vi "SelfParking.vi"() -> ()   [LabVIEW 2020]
uses:
  <vilib>/Instr/_visa.llb/VISA Flush IO Buffer Mask.ctl
  <vilib>/Instr/_visa.llb/VISA Configure Serial Port (Instr).vi
panel:
  out "Ask user":bool
  out "Perpendicular":bool
  out "Parallel":bool
  out "Execute":bool
  out "Move to stop line":bool
  out "Wait for start":bool
  out "Ask user":bool
  out "Scanning":bool
  out "String":string
  in  "module path":path
  in  "stop 2":bool
  in  "stop":bool
  out "Centimeters":i32
  in  "VISA resource name":refnum<visa-resource-name>
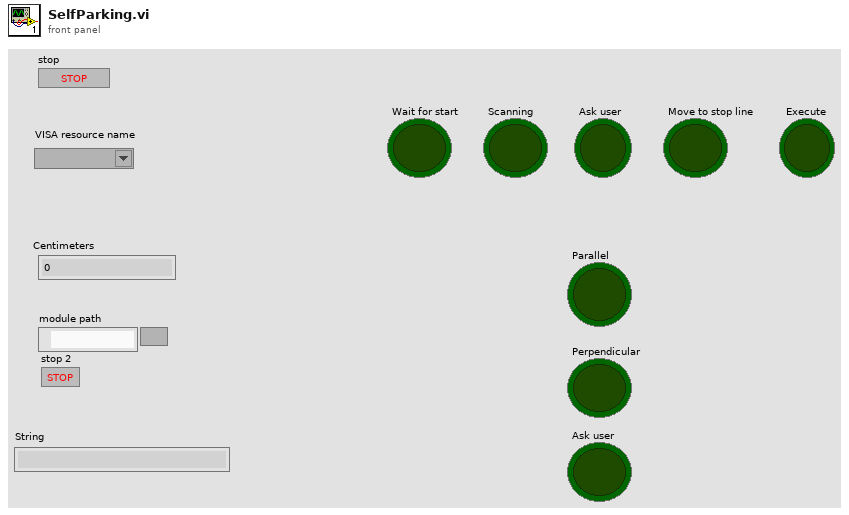
[diagram p1: front panel]
types:
  T1 = enum16{"wait for start", "move to stop line", "scanning", "ask user", "execute park"}
  T2 = typedef "VISA Flush IO Buffer Mask.ctl" = u16
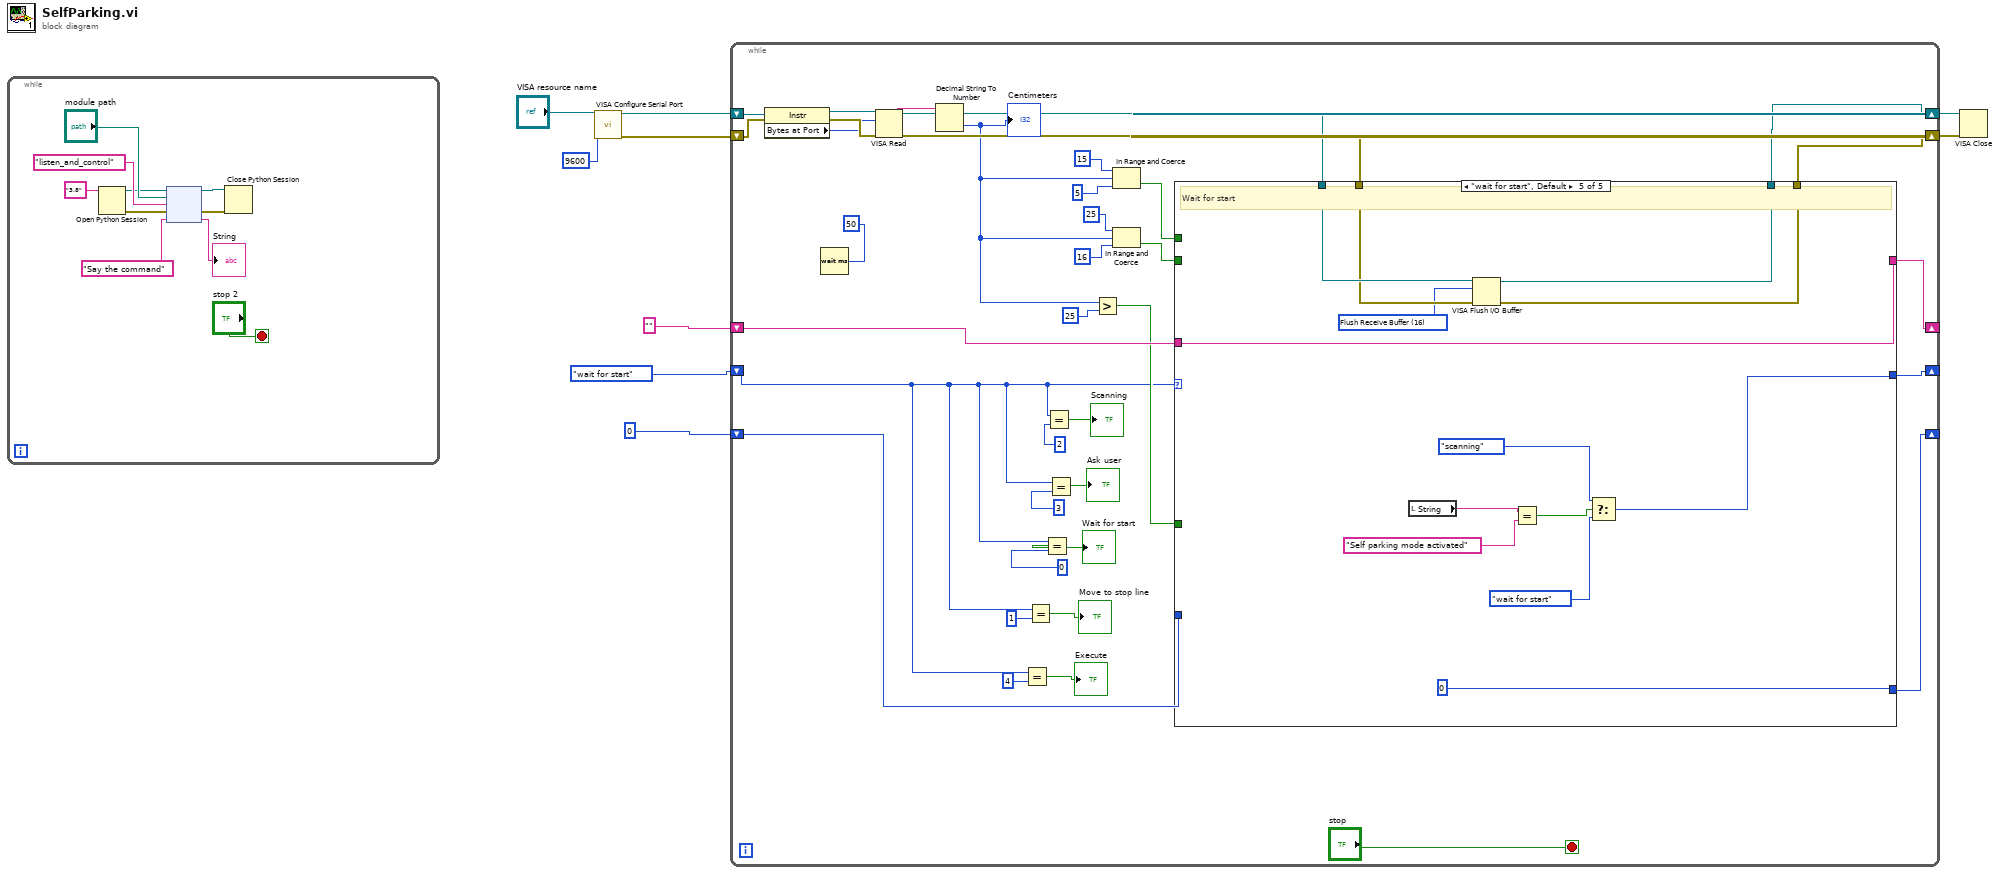
[diagram p0: block diagram]
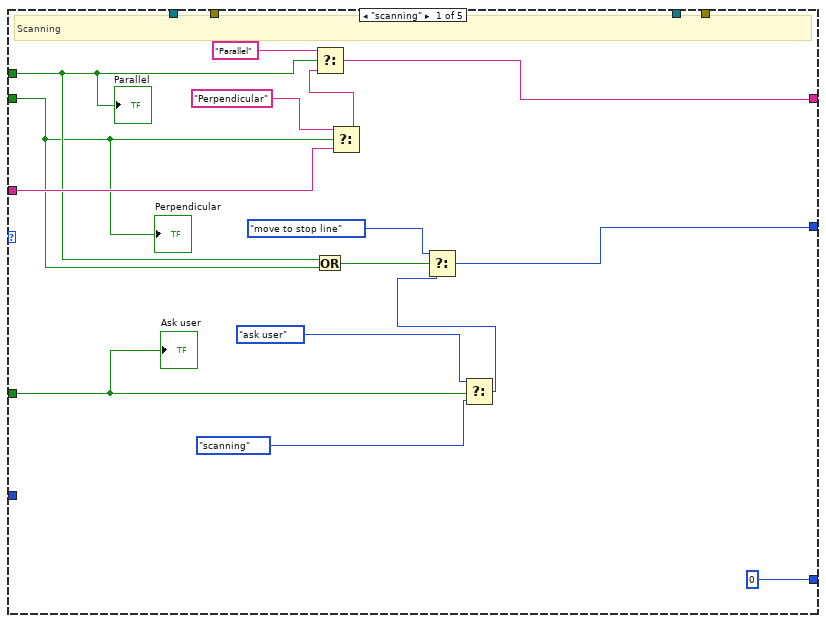
[diagram p2: hidden frame]
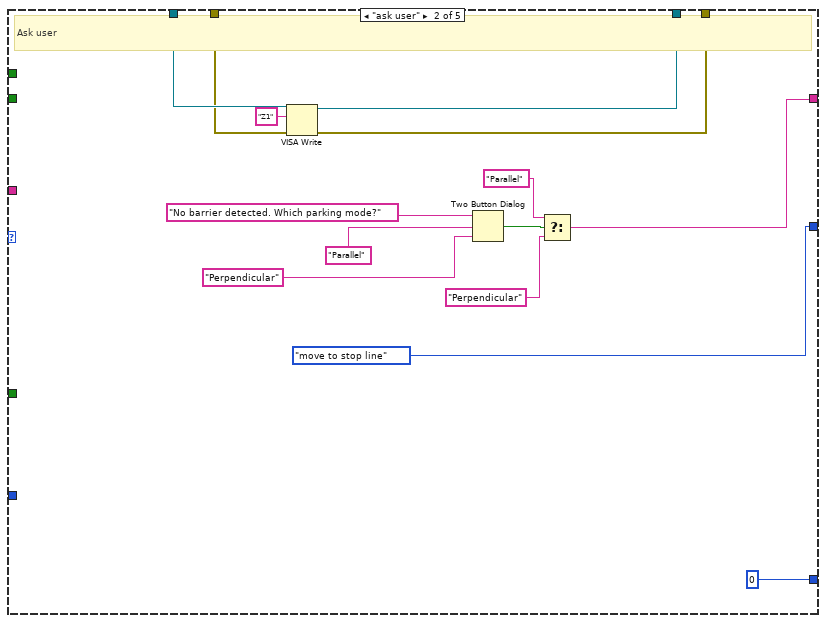
[diagram p3: hidden frame]
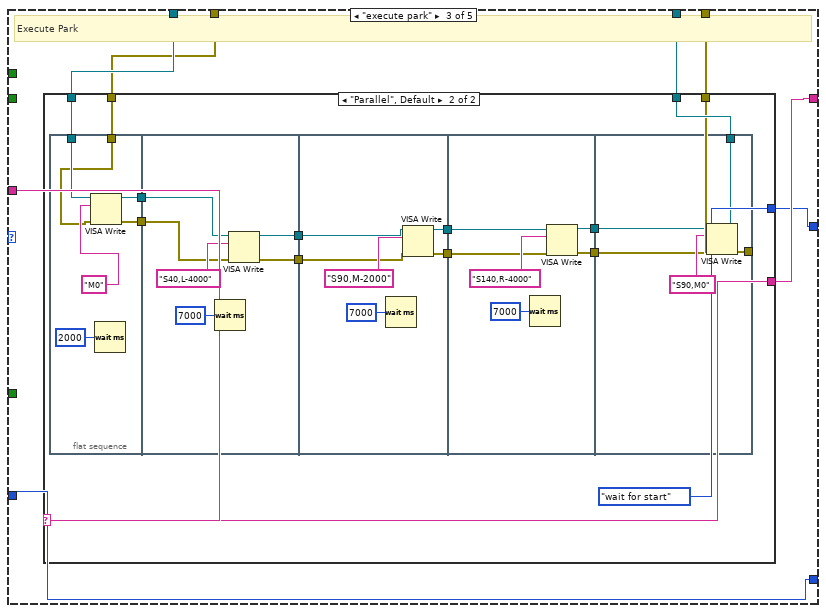
[diagram p4: hidden frame]
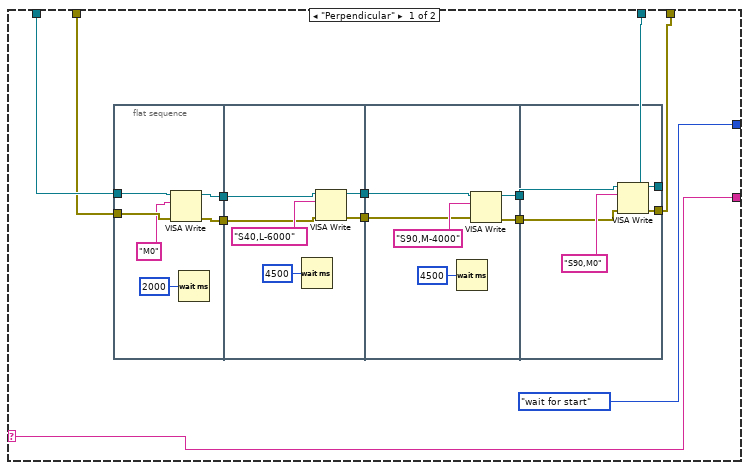
[diagram p5: hidden frame]
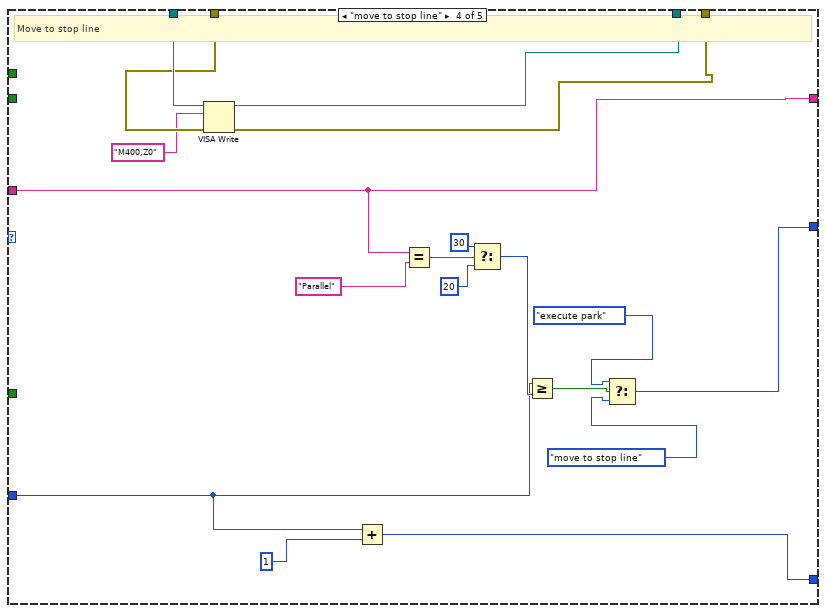
[diagram p6: hidden frame]
diagram:
  n1 = while {
    stop <- "stop 2" stop-if-true
    n2 = Open Python Session(python version="3.8" ("Python version")) -> (session out=w14:refnum<k35>, error out=w13:errorcluster)  [unwired: 2 in]
    n3 = node(w14, "module path", "listen_and_control" ("function name"), w13, "Say the command") -> (w15:refnum<k35>, w12:errorcluster, →"String":string)  [unwired: 2 out]
    n4 = Close Python Session(session in=w15, error in=w12) -> ()  [unwired: 1 out]
  }
  n5 = call-poly "VISA Configure Serial Port"("VISA resource name"="VISA resource name", "baud rate (9600)"=u32 9600) -> ("VISA resource name out"=w5:refnum<visa-resource-name>, "error out"=w4:errorcluster)  [unwired: 12 in]
  n6 = while {
    shift-right: [w40] -> w7
    shift-left: w5 -> [w53]
    shift-right: [w39] -> w6
    shift-left: w4 -> [w51]
    shift-right: [w46] -> _
    shift-left: 0 -> [w45]
    shift-right: [w43] -> _
    shift-left: "" -> [w44]
    shift-right: [w20] -> _
    shift-left: T1."wait for start" -> [w26]
    stop <- "stop" stop-if-true
    n7 = property class="Instr"(reference=w53, error in=w51) -> (reference out=w52:refnum<visa-resource-name>, error out=w50:errorcluster, "Bytes at Port"=w49:u32)
    n8 = Wait (ms)(milliseconds to wait=u32 50) -> ()  [unwired: 1 out]
    n9 = VISA Read(VISA resource name=w52, byte count=w49, error in (no error)=w50) -> (VISA resource name out=w41:refnum<visa-resource-name>, read buffer=w56:string, error out=w38:errorcluster)  [unwired: 1 out]
    n10 = Decimal String To Number(string=w56) -> (number=w21:i32)  [unwired: 2 in, 1 out]
    "Centimeters" <- w21
    n11 = Equal?(x=w26, y=u16 4) -> (x = y?=→"Execute":bool)
    n12 = Equal?(x=w26, y=u16 1) -> (x = y?=→"Move to stop line":bool)
    n13 = Equal?(x=w26, y=u16 0) -> (x = y?=→"Wait for start":bool)
    n14 = Equal?(x=w26, y=u16 2) -> (x = y?=→"Scanning":bool)
    n15 = Equal?(x=w26, y=u16 3) -> (x = y?=→"Ask user":bool)
    n16 = Greater?(x=w21, y=25) -> (0:w42:bool)
    n17 = In Range and Coerce(upper limit=15, x=w21, lower limit=5) -> (In Range?=w48:bool)  [unwired: 1 out]
    n18 = In Range and Coerce(upper limit=25, x=w21, lower limit=16) -> (In Range?=w47:bool)  [unwired: 1 out]
    n19 = case shown="\"wait for start\", Default" w26 {
      tunnel: w48 -> [w63 _ _ _ _]
      tunnel: w47 -> [w62 _ _ _ _]
      tunnel: [0 0 w94 w184 0] -> w46
      tunnel: w45 -> [_ _ w94 w186 _]
      tunnel: w44 -> [w70 _ w95 w191 w204]
      tunnel: [w68 w81 w89 w191 w204] -> w43
      tunnel: w42 -> [w61 _ _ _ _]
      tunnel: w41 -> [w66 w78 w93 w183 w196]
      tunnel: w38 -> [w65 w77 w92 w182 w194]
      tunnel: [w66 w75 w91 w181 w195] -> w40
      tunnel: [w65 w74 w90 w180 w193] -> w39
      tunnel: [w60 T1."move to stop line" w88 w178 w197] -> w20
      frame "scanning" {
        # "Scanning"
        n20 = Or(x=w63, y=w62) -> (x .or. y?=w71:bool)
        n21 = Select(t="Perpendicular", s=w62, f=w70) -> (s? t:f=w69:string)
        n22 = Select(t="Parallel", s=w63, f=w69) -> (s? t:f=w68:string)
        n23 = Select(t=T1."ask user", s=w61, f=T1."scanning") -> (s? t:f=w67:T1)
        n24 = Select(t=T1."move to stop line", s=w71, f=w67) -> (s? t:f=w60:T1)
        "Parallel" <- w63
        "Perpendicular" <- w62
        "Ask user" <- w61
      }
      frame "ask user" {
        # "Ask user"
        n25 = VISA Write(VISA resource name=w78, write buffer="Z1", error in (no error)=w77) -> (VISA resource name out=w75:refnum<visa-resource-name>, error out=w74:errorcluster)  [unwired: 1 out]
        n26 = Two Button Dialog(message="No barrier detected. Which parking mode?", 1:"Perpendicular" ("F button name (\"Cancel\")"), 2:"Parallel" ("T button name (\"OK\")")) -> (T button?=w84:bool)
        n27 = Select(t="Parallel", s=w84, f="Perpendicular") -> (s? t:f=w81:string)
      }
      frame "execute park" {
        # "Execute Park"
        n28 = case shown="\"Parallel\", Default" w95 {
          selector: w95 -> [w107 w144]
          tunnel: [w107 w144] -> w89
          tunnel: w93 -> [w106 w134]
          tunnel: w92 -> [w105 w133]
          tunnel: [T1."wait for start" T1."wait for start"] -> w88
          tunnel: [w100 w137] -> w91
          tunnel: [w99 w136] -> w90
          frame "Perpendicular" {
            n29 = flat-sequence {
              tunnel: w105 -> [w113]
              tunnel: w106 -> [w110]
              tunnel: [w112] -> w97
              tunnel: [w111] -> w96
              tunnel: [w117] -> w104
              tunnel: [w116] -> w103
              tunnel: w97 -> [w115]
              tunnel: w96 -> [w114]
              tunnel: w104 -> [w123]
              tunnel: w103 -> [w122]
              tunnel: [w121] -> w102
              tunnel: [w120] -> w101
              tunnel: w102 -> [w129]
              tunnel: w101 -> [w128]
              tunnel: [w127] -> w100
              tunnel: [w126] -> w99
              frame #0 {
                n30 = VISA Write(VISA resource name=w110, write buffer="M0", error in (no error)=w113) -> (VISA resource name out=w112:refnum<visa-resource-name>, error out=w111:errorcluster)  [unwired: 1 out]
                n31 = Wait (ms)(milliseconds to wait=u32 2000) -> ()  [unwired: 1 out]
              }
              frame #1 {
                n32 = Wait (ms)(milliseconds to wait=u32 4500) -> ()  [unwired: 1 out]
                n33 = VISA Write(VISA resource name=w115, write buffer="S40,L-6000", error in (no error)=w114) -> (VISA resource name out=w117:refnum<visa-resource-name>, error out=w116:errorcluster)  [unwired: 1 out]
              }
              frame #2 {
                n34 = Wait (ms)(milliseconds to wait=u32 4500) -> ()  [unwired: 1 out]
                n35 = VISA Write(VISA resource name=w123, write buffer="S90,M-4000", error in (no error)=w122) -> (VISA resource name out=w121:refnum<visa-resource-name>, error out=w120:errorcluster)  [unwired: 1 out]
              }
              frame #3 {
                n36 = VISA Write(VISA resource name=w129, write buffer="S90,M0", error in (no error)=w128) -> (VISA resource name out=w127:refnum<visa-resource-name>, error out=w126:errorcluster)  [unwired: 1 out]
              }
            }
          }
          frame "Parallel", Default {
            n37 = flat-sequence {
              tunnel: w134 -> [w148]
              tunnel: w133 -> [w147]
              tunnel: [w146] -> w132
              tunnel: [w145] -> w131
              tunnel: [w154] -> w143
              tunnel: [w153] -> w140
              tunnel: w132 -> [w152]
              tunnel: w131 -> [w151]
              tunnel: w143 -> [w160]
              tunnel: [w159] -> w142
              tunnel: w140 -> [w158]
              tunnel: [w157] -> w139
              tunnel: w142 -> [w166]
              tunnel: [w165] -> w141
              tunnel: w139 -> [w164]
              tunnel: [w163] -> w138
              tunnel: w141 -> [w172]
              tunnel: w138 -> [w171]
              tunnel: [w170] -> w137
              tunnel: [w169] -> w136
              frame #0 {
                n38 = VISA Write(VISA resource name=w148, write buffer="M0", error in (no error)=w147) -> (VISA resource name out=w146:refnum<visa-resource-name>, error out=w145:errorcluster)  [unwired: 1 out]
                n39 = Wait (ms)(milliseconds to wait=u32 2000) -> ()  [unwired: 1 out]
              }
              frame #1 {
                n40 = Wait (ms)(milliseconds to wait=u32 7000) -> ()  [unwired: 1 out]
                n41 = VISA Write(VISA resource name=w152, write buffer="S40,L-4000", error in (no error)=w151) -> (VISA resource name out=w154:refnum<visa-resource-name>, error out=w153:errorcluster)  [unwired: 1 out]
              }
              frame #2 {
                n42 = Wait (ms)(milliseconds to wait=u32 7000) -> ()  [unwired: 1 out]
                n43 = VISA Write(VISA resource name=w160, write buffer="S90,M-2000", error in (no error)=w158) -> (VISA resource name out=w159:refnum<visa-resource-name>, error out=w157:errorcluster)  [unwired: 1 out]
              }
              frame #3 {
                n44 = Wait (ms)(milliseconds to wait=u32 7000) -> ()  [unwired: 1 out]
                n45 = VISA Write(VISA resource name=w166, write buffer="S140,R-4000", error in (no error)=w164) -> (VISA resource name out=w165:refnum<visa-resource-name>, error out=w163:errorcluster)  [unwired: 1 out]
              }
              frame #4 {
                n46 = VISA Write(VISA resource name=w172, write buffer="S90,M0", error in (no error)=w171) -> (VISA resource name out=w170:refnum<visa-resource-name>, error out=w169:errorcluster)  [unwired: 1 out]
              }
            }
          }
        }
      }
      frame "move to stop line" {
        # "Move to stop line"
        n47 = VISA Write(VISA resource name=w183, write buffer="M400,Z0", error in (no error)=w182) -> (VISA resource name out=w181:refnum<visa-resource-name>, error out=w180:errorcluster)  [unwired: 1 out]
        n48 = Add(x=w186, y=1) -> (x+y=w184:i32)
        n49 = Equal?(x=w191, y="Parallel") -> (x = y?=w189:bool)
        n50 = Select(t=30, s=w189, f=20) -> (s? t:f=w188:i32)
        n51 = Greater Or Equal?(x=w186, y=w188) -> (x >= y?=w187:bool)
        n52 = Select(t=T1."execute park", s=w187, f=T1."move to stop line") -> (s? t:f=w178:T1)
      }
      frame "wait for start", Default {
        w192 = T2 16 items=["Flush Receive Buffer"=16, "Write Transmit Buffer to Device"=32, "Flush Receive Buffer (No I/O)"=64, "Flush Transmit Buffer"=128] ("Mask")
        # "Wait for start"
        n53 = local read "String"() -> (w199:string)
        n54 = VISA Flush I/O Buffer(VISA resource name=w196, mask (16)=w192, error in (no error)=w194) -> (VISA resource name out=w195:refnum<visa-resource-name>, error out=w193:errorcluster)
        n55 = Equal?(x=w199, y="Self parking mode activated") -> (x = y?=w198:bool)
        n56 = Select(t=T1."scanning", s=w198, f=T1."wait for start") -> (s? t:f=w197:T1)
      }
    }
  }
  n57 = VISA Close(VISA resource name=w7, error in (no error)=w6) -> ()  [unwired: 1 out]
